vi "Thermometer (Demo).vi"(7 "entrée d'erreur (pas d'erreur)":errorcluster, 9 "Échelle de temp.":bool) -> (0 "sortie d'erreur":errorcluster, 2 "Température":dbl(slide) scale=0.0..100.0 scale format="%.1f")   [LabVIEW 2009]
doc: "Ce VI simule la mesure d'une température sur le capteur intégré au boîtier de démonstration DAQ.\n\nSi vous disposez d'une carte DAQ et d'un boîtier de démonstration DAQ, alors utilisez plutôt le VI Thermometer."
panel:
  # "° C\n\n° F"
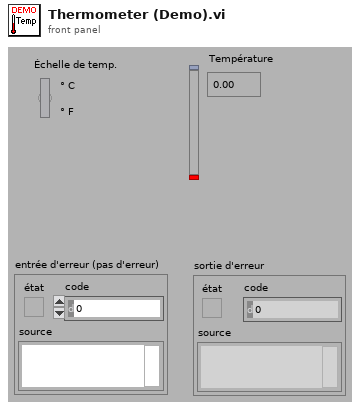
[diagram p1: front panel]
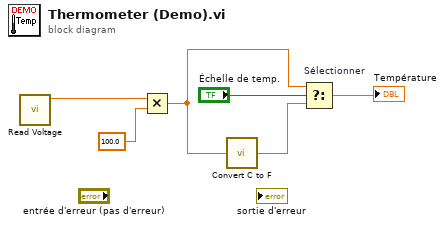
[diagram p0: block diagram]
diagram:
  n1 = call "Read Voltage.vi"() -> ("tension"=w1:dbl)  [unwired: 1 in, 6 out]
  n2 = Multiply ("Multiplier")(x=w1, y=100.0) -> (x*y=w2:dbl)
  n3 = call "Convert C to F.vi"("° C"=w2) -> ("° F"=w5:dbl)
  n4 = Select "Sélectionner"(t=w2, s="Échelle de temp.", f=w5) -> (s? t:f=→"Température":dbl)
